vi "PSCHN_Convert Cards To CHInfo.vi"(10 "Cards":T1[](array[typedef])) -> (2 "VCH":T3[](array[typedef]))   [LabVIEW 2016]
uses:
  DAQ-VirtualCH/SubVIs/VCH/Private/Ctrls/PSVCH_All Channels.ctl
  Controls/PSCHN_Card Para.ctl
  Controls/PSCHN_Channel Para.ctl
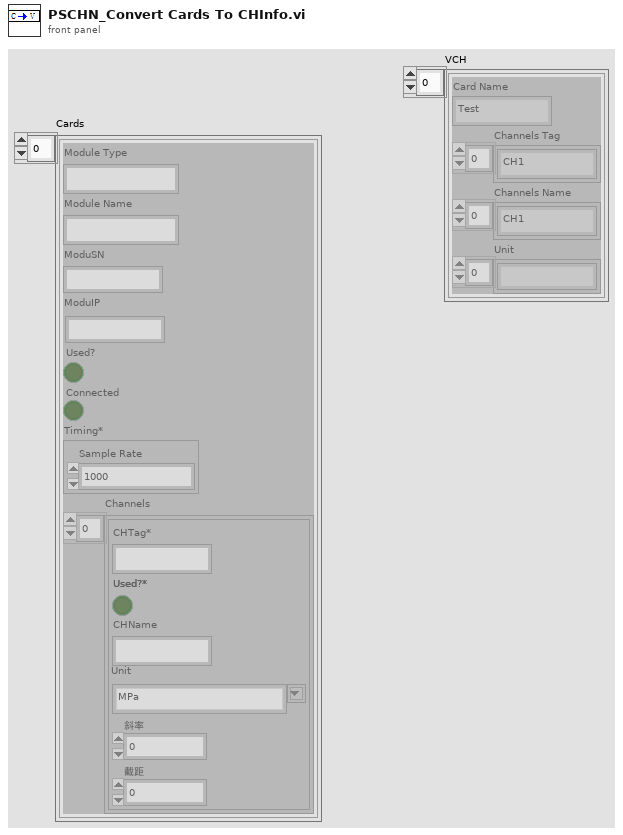
[diagram p1: front panel]
types:
  T1 = typedef "PSCHN_Card Para.ctl" = cluster{"Module Type":string, "Module Name":string, "ModuSN":string, "ModuIP":string, "Used?":bool, "Connected":bool, "Timing*":cluster{"Sample Rate":dbl}, "Channels":T2[]}
  T2 = typedef "PSCHN_Channel Para.ctl" = cluster{"CHTag*":string, "Used?*":bool, "CHName":string, "Unit":string, "斜率":dbl, "截距":dbl}
  T3 = typedef "PSVCH_All Channels.ctl" = cluster{"Card Name":string, "Channels Tag":string[], "Channels Name":string[], "Unit":string[]}
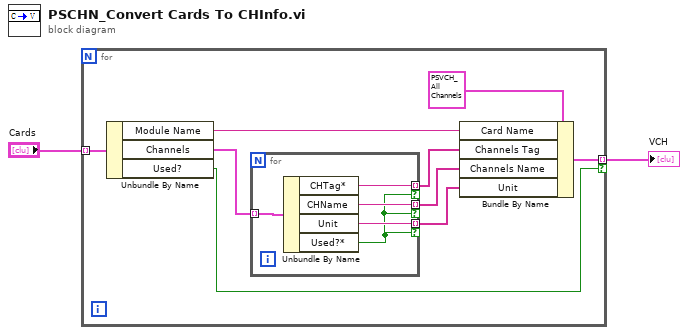
[diagram p0: block diagram]
diagram:
  n1 = for {
    tunnel: "Cards" -> [w11] mode=indexing
    tunnel: [w5] -> w1 mode=indexing if=w4
    n2 = Unbundle By Name(w11) -> ("Module Name"=w9:string, "Channels"=w10:T2[], "Used?"=w4:bool)
    n3 = for {
      tunnel: w10 -> [w16] mode=indexing
      tunnel: [w12] -> w6 mode=indexing if=w13
      tunnel: [w15] -> w8 mode=indexing if=w13
      tunnel: [w14] -> w7 mode=indexing if=w13
      n4 = Unbundle By Name(w16) -> ("CHTag*"=w12:string, "CHName"=w14:string, "Unit"=w15:string, "Used?*"=w13:bool)
    }
    n5 = Bundle By Name(cluster=T3 {"Card Name"="Test", "Channels Tag"=["CH1", "CH2"], "Channels Name"=["CH1", "CH2"], "Unit"=["", ""]} ("DAQ2ANA"), "Card Name"=w9, "Channels Tag"=w6, "Channels Name"=w7, "Unit"=w8) -> (w5:T3)
  }
  "VCH" <- w1
